vi "Create DIOs RT FIFO.vi"(8 "error in":errorcluster) -> (0 "error out":errorcluster, 3 "DIOs RT FIFO out":refnum<k33>)   [LabVIEW 2021, in "RT Main.lvlib"]
uses:
  RT Main.lvlib
  Libraries/Common Files/Common Files.lvlib
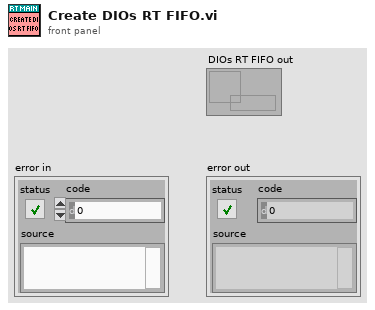
[diagram p1: front panel]
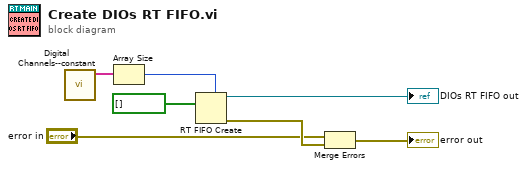
[diagram p0: block diagram]
diagram:
  n1 = call "Digital Channels--constant.vi"() -> ("Digital Channels--constant"=w4:tag[])  [unwired: 11 in]
  n2 = Array Size(array=w4) -> (size(s)=w1:i32)
  n3 = RT FIFO Create(1:bool[] [], 6:w1) -> (8:→"DIOs RT FIFO out":refnum<k33>, 11:w7:errorcluster)  [unwired: 6 in, 1 out]
  n4 = Merge Errors("error in", w7) -> (→"error out":errorcluster)
